vi "Mouse Reset.vi"(4 "Timeout (ms)":i32=100, 5 "FPGA VI Reference In":refnum<k20>) -> (0 "Timed out?":bool, 2 "FPGA VI Reference Out":refnum<k20>)   [LabVIEW 2012]
uses:
  <vilib>/Utility/error.llb/Error Cluster From Error Code.vi
  <vilib>/rvi/errors/niLvFpgaAdjustHostInterfaceError.vi
  <vilib>/rvi/interface/nirviReadWriteControl/nirviReadWriteControl.xnode
  NiFpgaLv.dll
  <vilib>/rvi/interface/Simulation/niFpgaSimulationCallBeginRW.vi
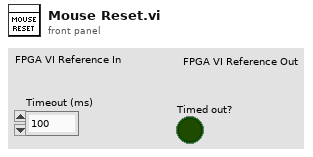
[diagram p1: front panel]
types:
  T1 = enum16{"idle", "set idle", "begin", "write", "read", "power down", "reset"}
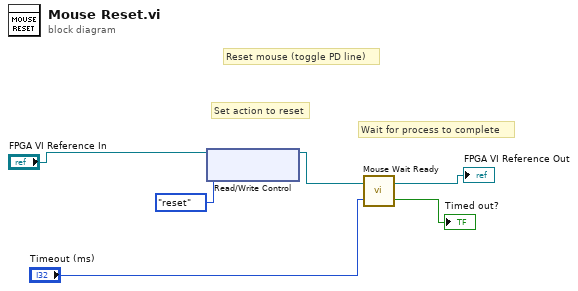
[diagram p0: block diagram]
diagram:
  # "Wait for process to complete"
  # "Set action to reset"
  # "Reset mouse (toggle PD line)"
  n1 = xnode "Read/Write Control"("FPGA VI Reference In"="FPGA VI Reference In", "Mouse Action"=T1."reset") -> ("FPGA VI Reference Out"=w4:refnum<k20>)  [unwired: 1 in, 1 out]
  n2 = call "Mouse Wait Ready.vi"("Timeout (ms)"="Timeout (ms)", "Refnum in"=w4) -> ("Timeout"=→"Timed out?":bool, "Refnum out"=→"FPGA VI Reference Out":refnum<k20>)
